vi "LabVIEWWebsocketChart - Multiple Connection.vi"() -> ()   [LabVIEW 2014]
uses:
  Modules/Library/Method.ctl
  <vilib>/myRIO/Instrument Drivers/Onboard IO/DIO/typedefs/DIO Reference.ctl
  <vilib>/myRIO/Common/Instrument Driver Framework/Utilities/typedefs/myRIO Generic Hardware Reference.ctl
  <vilib>/myRIO/Common/Instrument Driver Framework/Utilities/typedefs/Hardware Version Enum.ctl
  <vilib>/myRIO/Common/Instrument Driver Framework/Utilities/typedefs/myRIO v1.0 Reference.ctl
  <vilib>/myRIO/Common/Instrument Driver Framework/Utilities/typedefs/Generic FPGA Reference.ctl
  <vilib>/myRIO/Common/Instrument Driver Framework/myRIO v1.0/DIO/typedefs/DIO Channels List.ctl
  <vilib>/myRIO/Common/Instrument Driver Framework/myRIO v1.0/DIO/typedefs/DIO Channels Enum.ctl
  <vilib>/userdefined/High Color/nirio_resource_hc.ctl
  Modules/Library/Connection.ctl
  <vilib>/NI/STM/SubVIs/MetaDataElement.ctl
  <vilib>/myRIO/Instrument Drivers/Onboard Devices/Accelerometer/typedefs/Accelerometer Reference.ctl
  <vilib>/myRIO/Common/Instrument Driver Framework/myRIO v1.0/Accelerometer/typedefs/Accelerometer Channels List.ctl
  <vilib>/myRIO/Common/Instrument Driver Framework/myRIO v1.0/Accelerometer/typedefs/Accelerometer Channels Enum.ctl
  <vilib>/myRIO/Common/Instrument Driver Framework/Utilities/vis/Is FPGA Ref Available.vi
  <vilib>/myRIO/Common/Instrument Driver Framework/myRIO v1.0/DIO/vis/myRIO v1.1 Open DIO.vi
  <vilib>/myRIO/Instrument Drivers/Onboard IO/DIO/vis/Read.vi
  <vilib>/myRIO/Common/Instrument Driver Framework/myRIO v1.0/Accelerometer/vis/myRIO v1.1 Open Accelerometer.vi
  <vilib>/myRIO/Instrument Drivers/Onboard Devices/Accelerometer/vis/Read.vi
  <vilib>/myRIO/Instrument Drivers/Onboard IO/DIO/vis/Write.vi
  <vilib>/myRIO/Common/Instrument Driver Framework/Utilities/vis/Validate Channels.vi
  <vilib>/myRIO/Common/Instrument Driver Framework/myRIO v1.0/DIO/vis/myRIO v1.0 Reserve DIO.vi
  <vilib>/myRIO/Common/Instrument Driver Framework/myRIO v1.0/Accelerometer/vis/myRIO v1.0 Reserve Accelerometer.vi
  <vilib>/myRIO/Common/Instrument Driver Framework/myRIO v1.0/Resource Manager/vis/myRIO v1.0 Reserve Channel List.vi
  <vilib>/myRIO/Common/Instrument Driver Framework/myRIO v1.0/DIO/vis/myRIO v1.0 Build MUX Configuration DIO.vi
  <vilib>/myRIO/Common/Instrument Driver Framework/myRIO v1.0/Accelerometer/vis/myRIO v1.0 Build MUX Configuration Accelerometer.vi
  <vilib>/myRIO/Common/Instrument Driver Framework/myRIO v1.0/Resource Manager/vis/myRIO v1.0 Reserve Channel.vi
  <vilib>/myRIO/Common/Instrument Driver Framework/myRIO v1.0/Resource Manager/vis/myRIO v1.0 Unreserve Channel.vi
  <vilib>/myRIO/Common/Instrument Driver Framework/myRIO v1.0/Resource Manager/vis/myRIO v1.0 Create Configuration List.vi
  <vilib>/myRIO/Common/Instrument Driver Framework/myRIO v1.0/Resource Manager/vis/myRIO v1.0 Build Mutex Name.vi
  <vilib>/Utility/VariantDataType/GetNumericInfo.vi
  <vilib>/Utility/error.llb/Error Cluster From Error Code.vi
  <vilib>/myRIO/Common/Instrument Driver Framework/myRIO v1.0/myRIO v1.1 Open.vi
  <vilib>/myRIO/Common/Instrument Driver Framework/Utilities/vis/IO Manager.vi
  <vilib>/myRIO/Common/Instrument Driver Framework/Utilities/vis/Configuration Manager.vi
  <vilib>/myRIO/Common/Instrument Driver Framework/myRIO v1.0/Resource Manager/vis/myRIO v1.0 Configure IO.vi
  <vilib>/myRIO/Common/Instrument Driver Framework/myRIO v1.0/myRIO v1.0 Close.vi
  <vilib>/myRIO/Common/Instrument Driver Framework/myRIO v1.0/DIO/vis/myRIO v1.0 Read DIO.vi
  <vilib>/functionblocks/Edge Detection/One Shot Rising with Input/One Shot Rising with Input.vi
  <vilib>/myRIO/Common/Instrument Driver Framework/myRIO v1.0/DIO/vis/myRIO v1.0 Write DIO.vi
  <vilib>/myRIO/Common/Instrument Driver Framework/myRIO v1.0/Accelerometer/vis/myRIO v1.0 Get Scaling Constant Accelerometer.vi
  <vilib>/myRIO/Common/Instrument Driver Framework/myRIO v1.0/Accelerometer/vis/myRIO v1.0 Read Accelerometer.vi
  <vilib>/myRIO/Express VI/Onboard Devices/Button/Button Express VI.xnode
  <vilib>/myRIO/Instrument Drivers/Onboard IO/DIO/vis/myRIO DIO Open.xnode
  <vilib>/functionblocks/FB Core/FB Core.xnode
  <vilib>/myRIO/Express VI/Onboard Devices/LED/LED Express VI.xnode
  <vilib>/myRIO/Express VI/Onboard Devices/Accelerometer/Accelerometer Express VI.xnode
  <vilib>/myRIO/Instrument Drivers/Onboard Devices/Accelerometer/vis/myRIO Accelerometer Open.xnode
  <vilib>/Intelligent Energy/WebSockets API/WebSockets/WebSockets.lvlib
  <vilib>/NI/STM/NI STM.lvlib
  <vilib>/myRIO/Instrument Drivers/Onboard IO/DIO/DIO.lvlib
  <vilib>/functionblocks/NI_FunctionBlock Libraries.lvlib
  <vilib>/myRIO/Instrument Drivers/Onboard Devices/Accelerometer/Accelerometer.lvlib
panel:
  out "Chart":T1(graph)
  out "LED 2":bool
  out "LED 1":bool
  out "User Text (Log)":string="\r\n"
  out "User Text (Last)":string
  out "data (default)":string
  out "msg (default)":string="ssssss"
  out "data (JSON) 2":string
  out "msg (string)":string="Core : CN Close"
  in  "Toggle LED 2":bool
  in  "Toggle LED 1":bool
  out "Request URI":string="/"
  out "HTTP Headers":variant=variant("Accept"=variant(string "text/html,application/xhtml+xml,application/xml;q=0.9,*/*;q=0.8"), "Accept-Encoding"=variant(string "gzip, deflate"), "Accept-Language"=variant(string "en-GB,en;q=0.5"), "Cache-Control"=variant(string "no-cache"), "Connection"=variant(string "keep-alive, Upgrade"), "DNT"=variant(string "1"), "Host"=variant(string "localhost:6125"), "Origin"=variant(string "http://localhost:8000"), "Pragma"=variant(string "no-cache"), "Sec-WebSocket-Extensions"=variant(string "permessage-deflate"), "Sec-WebSocket-Key"=variant(string "dPMfcRTFpHjstnxySTdG7A=="), "Sec-WebSocket-Version"=variant(string "13"), "Upgrade"=variant(string "websocket"), "User-Agent"=variant(string "Mozilla/5.0 (Windows NT 10.0; WOW64; rv:42.0) Gecko/20100101 Firefox/42.0"))
  in  "Stop":bool
  in  "Send":bool
  in  "Message":string="new message"
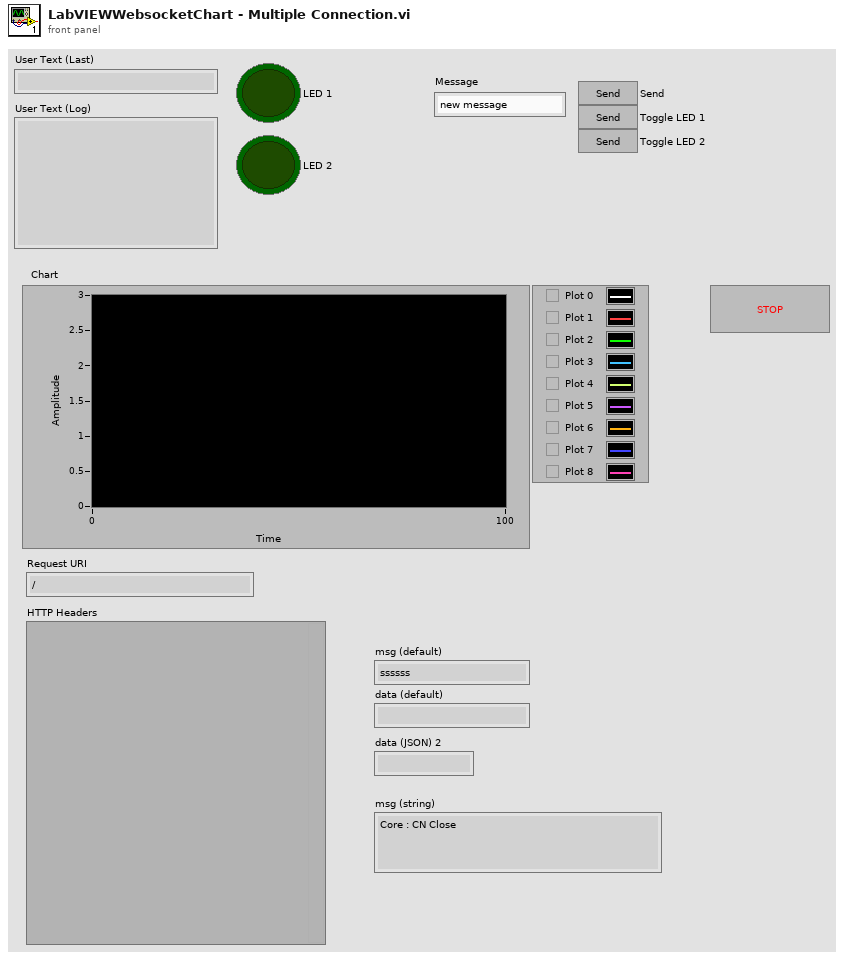
[diagram p1: front panel]
types:
  T1 = cluster{"[0]":dbl, "[1]":dbl, "[2]":dbl, "[3]":dbl, "[4]":dbl, "[5]":dbl, "[6]":dbl, "[7]":dbl, "[8]":dbl}
  T2 = typedef "Method.ctl" = enum16{"Initialize", "Add Connection", "Set Properties", "Get Connection(s)", "Remove Connection", "Remove All Connections", "Get Connection Count"}
  T3 = typedef "DIO.lvlib/DIO Reference.ctl" = cluster{"myRIO Reference":T4, "DIO Channels List":T8}
  T4 = typedef "myRIO Generic Hardware Reference.ctl" = cluster{"myRIO Model":T5, "myRIO Hardware Reference":T6}
  T5 = typedef "Hardware Version Enum.ctl" = enum16{"Unknown", "myRIO-1900", "myRIO-1950"}
  T6 = typedef "myRIO v1.0 Reference.ctl" = cluster{"Generic FPGA Reference":T7, "Allow multiple opens":bool}
  T7 = typedef "Generic FPGA Reference.ctl" = refnum<k20>
  T8 = typedef "DIO Channels List.ctl" = T9[]
  T9 = typedef "DIO Channels Enum.ctl" = enum16{"Not Connected", "C/DIO0", "C/DIO1", "C/DIO2", "C/DIO3", "C/DIO4", "C/DIO5", "C/DIO6", "C/DIO7", "A/DIO0", "A/DIO1", "A/DIO2", "A/DIO3", "A/DIO4", "A/DIO5", "A/DIO6", "A/DIO7", "A/DIO8", "A/DIO9", "A/DIO10", "A/DIO11", "A/DIO12", "A/DIO13", "A/DIO14", "A/DIO15", "B/DIO0", "B/DIO1", "B/DIO2", "B/DIO3", "B/DIO4", "B/DIO5", "B/DIO6", "B/DIO7", "B/DIO8", "B/DIO9", "B/DIO10", "B/DIO11", "B/DIO12", "B/DIO13", "B/DIO14", "B/DIO15", "LED0", "LED1", "LED2", "LED3", "Button0"}
  T10 = typedef "nirio_resource_hc.ctl" = tag
  T11 = typedef "NI STM.lvlib/TCP Connection Info.ctl" = cluster{"connection ID":refnum<k5>, "meta data":T12[]}
  T12 = typedef "NI STM.lvlib/MetaDataElement.ctl" = string
  T13 = typedef "Connection.ctl" = cluster{"connection ID":refnum<k5>, "meta data":T12[]}
  T14 = typedef "Accelerometer.lvlib/Accelerometer Reference.ctl" = cluster{"myRIO Reference":T4, "Accelerometer Channels List":T15, "LSB Weight":dbl}
  T15 = typedef "Accelerometer Channels List.ctl" = T16[]
  T16 = typedef "Accelerometer Channels Enum.ctl" = enum16{"Not Connected", "X-Axis", "Y-Axis", "Z-Axis"}
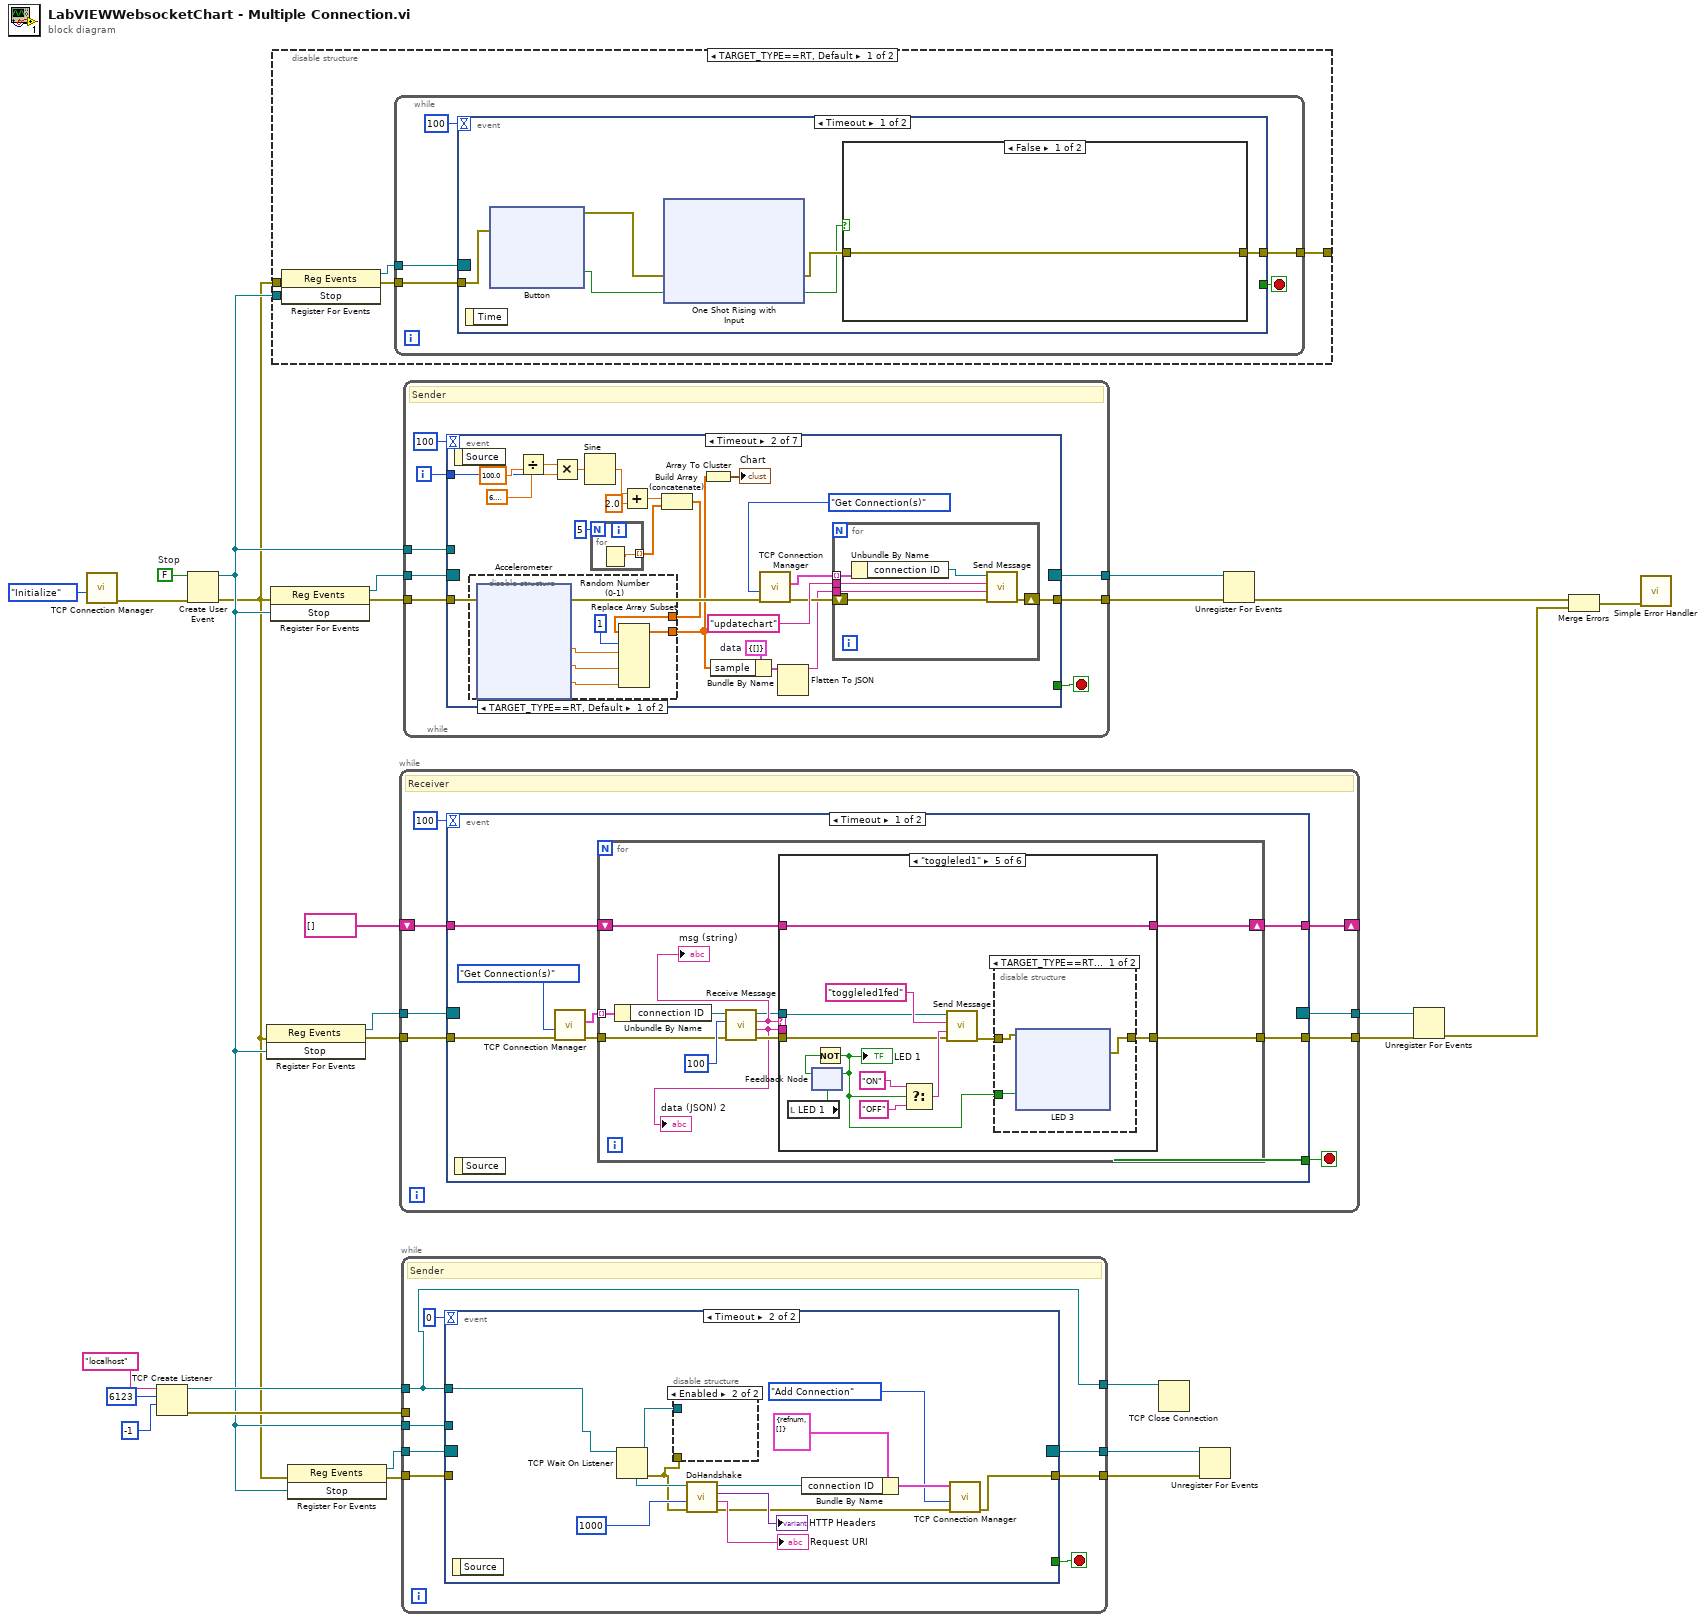
[diagram p0: block diagram]
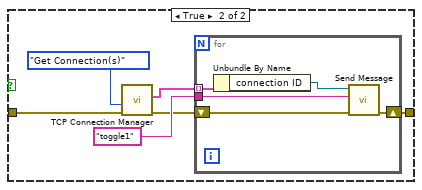
[diagram p2: hidden frame]
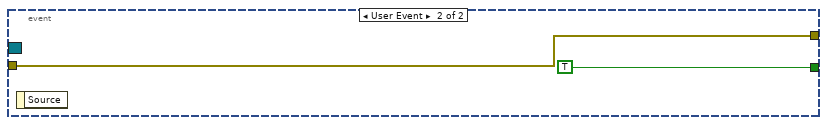
[diagram p3: hidden frame]
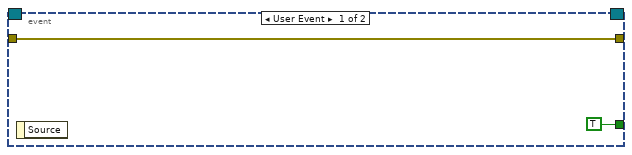
[diagram p5: hidden frame]
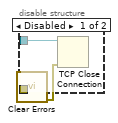
[diagram p6: hidden frame]
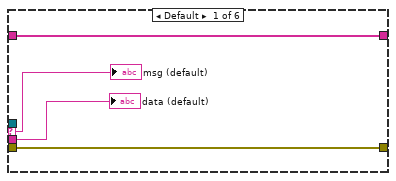
[diagram p7: hidden frame]
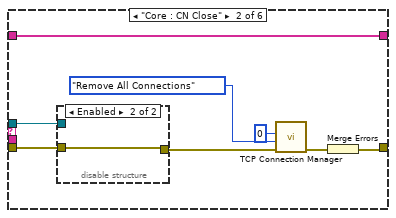
[diagram p8: hidden frame]
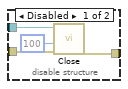
[diagram p9: hidden frame]
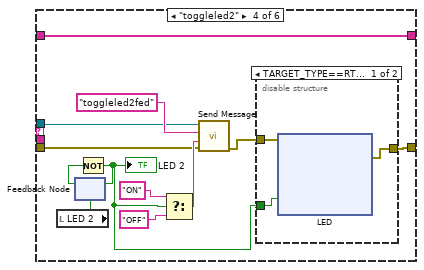
[diagram p11: hidden frame]
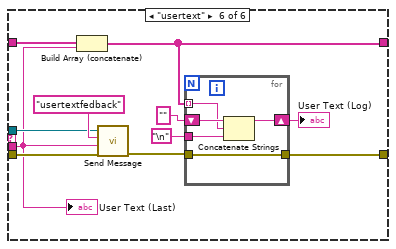
[diagram p14: hidden frame]
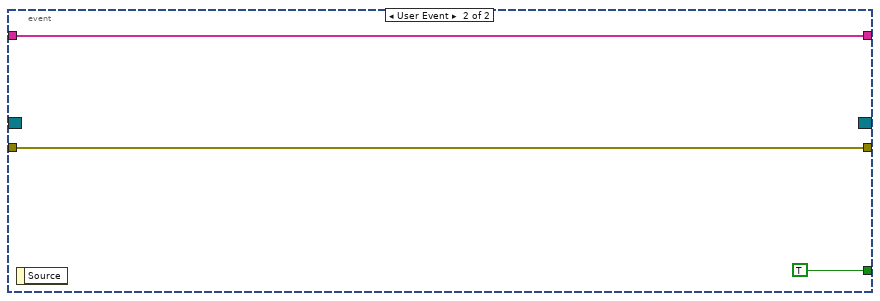
[diagram p15: hidden frame]
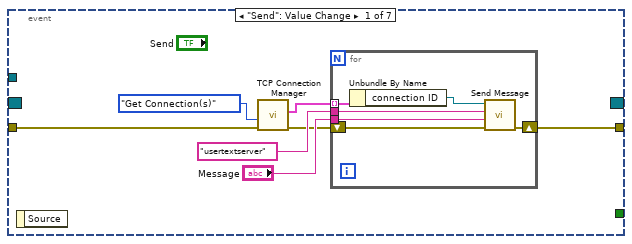
[diagram p16: hidden frame]
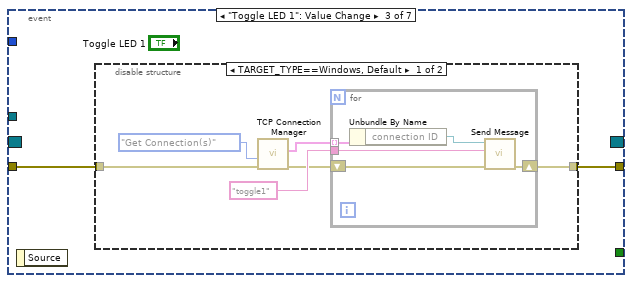
[diagram p18: hidden frame]
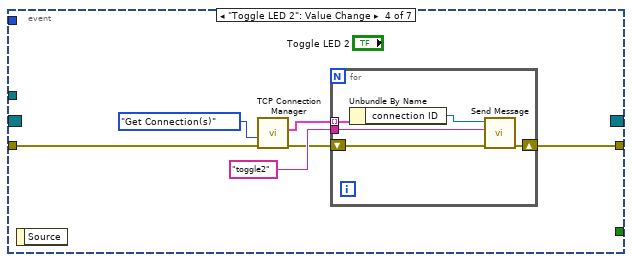
[diagram p20: hidden frame]
diagram:
  w27 = FALSE  # Stop
  n1 = call "TCP Connection Manager.vi"("method"=Method."Initialize") -> ("error out"=w10:errorcluster)  [unwired: 7 in, 3 out]
  n2 = TCP Create Listener(9:-1 ("timeout ms (25000)"), 10:u16 6123 ("port"), 11:"localhost" ("service name")) -> (0:w3:errorcluster, 3:w5:refnum<k5>)  [unwired: 2 in, 1 out]
  n3 = Create User Event(user event datatype=w27, error in=w10) -> (user event=w2:refnum<user-event>, error out=w1:errorcluster)
  n4 = register-events(error in=w1, w2) -> (reference out=w20:refnum<event-registration>, error out=w19:errorcluster)  [unwired: 1 in]
  n5 = register-events(error in=w1, w2) -> (reference out=w25:refnum<event-registration>, error out=w26:errorcluster)  [unwired: 1 in]
  n6 = disable-structure shown="TARGET_TYPE==RT, Default" {
    disable-tunnel: w2 -> [w31 _]
    disable-tunnel: w1 -> [w30 _]
    disable-tunnel: [w28 _] -> _
    frame condition #0 (active) {
      n7 = register-events(error in=w30, w31) -> (reference out=w29:refnum<event-registration>, error out=w32:errorcluster)  [unwired: 1 in]
      n8 = while {
        tunnel: w32 -> [w36]
        tunnel: w29 -> [w35]
        tunnel: [w33] -> w28
        stop <- w34 stop-if-true
        n9 = event shown="[0] Timeout" {
          selector: w35 -> [_ _]
          dyn-events: _ -> [_ _]
          timeout: 100 -> [_ _]
          tunnel: w36 -> [w42 w129]
          tunnel: [_ TRUE] -> w34
          tunnel: [w43 w129] -> w33
          event Timeout {
            n10 = event-data() -> ()  [unwired: 1 in, 1 out]
            n11 = xnode "Button"("error in (no error)"=w42) -> ("Value"=w40:bool, "error out"=w41:errorcluster)
            n12 = xnode "One Shot Rising with Input"("error in"=w41, "input"=w40) -> ("error out"=w39:errorcluster, "output"=w38:bool)
            n13 = case shown="False" w38 {
              tunnel: w39 -> [w117 w119]
              tunnel: [w117 w118] -> w43
              frame False {
              }
              frame True {
                n14 = call "TCP Connection Manager.vi"("error in"=w119, "method"=Method."Get Connection(s)") -> ("error out"=w122:errorcluster, "all connections"=w120:T11[])  [unwired: 6 in, 2 out]
                n15 = for {
                  tunnel: "toggle1" ("msg (string)") -> [w128]
                  tunnel: w120 -> [w126] mode=indexing
                  shift-right: [w124] -> w118
                  shift-left: w122 -> [w127]
                  n16 = Unbundle By Name(w126) -> ("connection ID"=w125:refnum<k5>)
                  n17 = call "Send Message.vi"("error in (no error)"=w127, "msg (string)"=w128, "WebSocket Connection in"=w125) -> ("error out"=w124:errorcluster)  [unwired: 7 in, 1 out]
                }
              }
            }
          }
          event User Event {
            n18 = event-data() -> ()  [unwired: 1 in, 1 out]
          }
        }
      }
    }
    frame condition #1 {
    }
  }
  n19 = register-events(error in=w1, w2) -> (reference out=w13:refnum<event-registration>, error out=w14:errorcluster)  [unwired: 1 in]
  n20 = while {
    tunnel: w20 -> [w136]
    tunnel: [w134] -> w22
    shift-right: [w131] -> _
    shift-left: string[] [] ("appended array") -> [w132]
    tunnel: w19 -> [w135]
    tunnel: [w137] -> w21
    stop <- w138 stop-if-true
    # "Receiver"
    n21 = event shown="[0] Timeout" {
      selector: w136 -> [_ _]
      dyn-events: [_ _] -> w134
      timeout: 100 -> [_ _]
      tunnel: [_ TRUE] -> w138
      tunnel: [w142 w295] -> w137
      tunnel: w135 -> [w145 w295]
      tunnel: w132 -> [w141 w294]
      tunnel: [w140 w294] -> w131
      event Timeout {
        n22 = event-data() -> ()  [unwired: 1 in, 1 out]
        n23 = call "TCP Connection Manager.vi"("error in"=w145, "method"=Method."Get Connection(s)") -> ("error out"=w143:errorcluster, "all connections"=w139:T11[])  [unwired: 6 in, 2 out]
        n24 = for {
          tunnel: w143 -> [w155]
          tunnel: [w151] -> w142
          tunnel: w139 -> [w154] mode=indexing
          shift-right: [w149] -> w140
          shift-left: w141 -> [w150]
          n25 = Unbundle By Name(w154) -> ("connection ID"=w153:refnum<k5>)
          n26 = call "Receive Message.vi"("error in (no error)"=w155, "timeout ms (5000)"=100, "WebSocket Connection in"=w153) -> ("error out"=w152:errorcluster, "data (JSON)"=w147:string, "msg (string)"=w148:string, "WebSocket Connection out"=w146:refnum<k5>)  [unwired: 5 in]
          "msg (string)" <- w148
          "data (JSON) 2" <- w147
          n27 = case shown="\"toggleled1\"" w148 {
            selector: w148 -> [w159 _ _ _ _ _]
            tunnel: w152 -> [w160 w167 w174 w181 w232 w286]
            tunnel: w147 -> [w158 _ _ _ _ w284]
            tunnel: [w160 w165 w174 w178 w228 w280] -> w151
            tunnel: w150 -> [w157 w168 w175 w180 w231 w288]
            tunnel: [w157 w168 w175 w180 w231 w278] -> w149
            tunnel: w146 -> [_ w166 _ w179 w230 w285]
            frame Default {
              "msg (default)" <- w159
              "data (default)" <- w158
            }
            frame "Core : CN Close" {
              n28 = disable-structure shown="Enabled" {
                disable-tunnel: w167 -> [w172 w173]
                disable-tunnel: w166 -> [w171 _]
                disable-tunnel: [w169 w173] -> w162
                frame Disabled {
                  n29 = call <vilib>:"Close.vi"("error in (no error)"=w172, "timeout ms (5000)"=100, "WebSocket Connection in"=w171) -> ("error out"=w169:errorcluster)  [unwired: 7 in, 1 out]
                }
                frame Enabled {
                }
              }
              n30 = call "TCP Connection Manager.vi"("error in"=w162, "method"=Method."Remove All Connections", "index"=0) -> ("error out"=w164:errorcluster)  [unwired: 5 in, 3 out]
              n31 = Merge Errors(w164) -> (w165:errorcluster)
            }
            frame "Core :Timeout" {
            }
            frame "toggleled2" {
              n32 = local read "LED 2"() -> (w182:bool)
              n33 = feedback #1(w182) -> (w183:bool)
              n34 = Not(x=w183) -> (.not. x?=w176:bool)
              "LED 2" <- w176
              n35 = feedback-in #1(w176) -> ()
              n36 = Select(t="ON", s=w176, f="OFF") -> (s? t:f=w187:string)
              n37 = call "Send Message.vi"("error in (no error)"=w181, "data (JSON)"=w187, "msg (string)"="toggleled2fed", "WebSocket Connection in"=w179) -> ("error out"=w177:errorcluster)  [unwired: 6 in, 1 out]
              n38 = disable-structure shown="TARGET_TYPE==RT, Default" {
                disable-tunnel: w177 -> [w190 w226]
                disable-tunnel: [w189 w226] -> w178
                disable-tunnel: w176 -> [w188 _]
                frame condition #0 (active) {
                  n39 = xnode "LED"("LED1"=w188, "error in (no error)"=w190) -> ("error out"=w189:errorcluster)
                }
                frame condition #1 {
                }
              }
            }
            frame "toggleled1" {
              n40 = local read "LED 1"() -> (w233:bool)
              n41 = feedback #2(w233) -> (w234:bool)
              n42 = Not(x=w234) -> (.not. x?=w227:bool)
              "LED 1" <- w227
              n43 = feedback-in #2(w227) -> ()
              n44 = Select(t="ON", s=w227, f="OFF") -> (s? t:f=w238:string)
              n45 = call "Send Message.vi"("error in (no error)"=w232, "data (JSON)"=w238, "msg (string)"="toggleled1fed", "WebSocket Connection in"=w230) -> ("error out"=w229:errorcluster)  [unwired: 6 in, 1 out]
              n46 = disable-structure shown="TARGET_TYPE==RT, Default" {
                disable-tunnel: w229 -> [w241 w277]
                disable-tunnel: [w240 w277] -> w228
                disable-tunnel: w227 -> [w239 _]
                frame condition #0 (active) {
                  n47 = xnode "LED 3"("LED0"=w239, "error in (no error)"=w241) -> ("error out"=w240:errorcluster)
                }
                frame condition #1 {
                }
              }
            }
            frame "usertext" {
              n48 = Build Array (concatenate)(w288, w284) -> (w278:string[])
              n49 = call "Send Message.vi"("error in (no error)"=w286, "data (JSON)"=w284, "msg (string)"="usertextfedback", "WebSocket Connection in"=w285) -> ("error out"=w279:errorcluster)  [unwired: 6 in, 1 out]
              n50 = for {
                tunnel: w278 -> [w291] mode=indexing
                shift-right: [w293] -> w282
                shift-left: "" -> [w292]
                tunnel: "\n" -> [w290]
                tunnel: w279 -> [w289]
                tunnel: [w289] -> w280
                n51 = Concatenate Strings(w292, w291, w290) -> (w293:string)
              }
              "User Text (Log)" <- w282
              "User Text (Last)" <- w284
            }
          }
        }
      }
      event User Event {
        n52 = event-data() -> ()  [unwired: 1 in, 1 out]
      }
    }
  }
  n53 = while {
    tunnel: w13 -> [w302]
    tunnel: [w300] -> w11
    tunnel: w2 -> [w299]
    tunnel: w14 -> [w301]
    tunnel: [w303] -> w12
    tunnel: w5 -> [w297]
    tunnel: [w297] -> w4
    tunnel: w3 -> [_]
    stop <- w304 stop-if-true
    # "Sender"
    n54 = event shown="[1] Timeout" {
      selector: w302 -> [_ _]
      dyn-events: [_ _] -> w300
      timeout: 0 -> [_ _]
      tunnel: [TRUE _] -> w304
      tunnel: [w305 w319] -> w303
      tunnel: w301 -> [w305 _]
      tunnel: w299 -> [_ _]
      tunnel: w297 -> [_ w307]
      event User Event {
        n55 = event-data() -> ()  [unwired: 1 in, 1 out]
      }
      event Timeout {
        n56 = event-data() -> ()  [unwired: 1 in, 1 out]
        n57 = TCP Wait On Listener(11:w307) -> (0:w308:errorcluster, 3:w309:refnum<k5>, 4:w315:refnum<k5>)  [unwired: 3 in, 2 out]
        n58 = disable-structure shown="Enabled" {
          disable-tunnel: w309 -> [w322 _]
          disable-tunnel: w308 -> [w321 _]
          frame Disabled {
            n59 = call <vilib>:"Clear Errors.vi"("error in (no error)"=w321) -> ("error out"=w320:errorcluster)  [unwired: 5 in, 1 out]
            n60 = TCP Close Connection(connection ID=w322, error in (no error)=w320) -> ()  [unwired: 1 in, 2 out]
          }
          frame Enabled {
          }
        }
        n61 = call <vilib>:"DoHandshake.vi"("error in (no error)"=w308, "timeout ms (5000)"=1000 ("timeout ms (25000)"), "WebSocket Connection in"=w315) -> ("error out"=w312:errorcluster, "Request URI"=→"Request URI":string, "Headers Out"=→"HTTP Headers":variant, "WebSocket Connection out"=w313:refnum<k5>)  [unwired: 5 in]
        n62 = Bundle By Name(cluster=T13 {"connection ID"=refnum, "meta data"=[]} ("connection in"), "connection ID"=w313) -> (w311:T13)
        n63 = call "TCP Connection Manager.vi"("error in"=w312, "method"=Method."Add Connection", "connection in"=w311) -> ("error out"=w319:errorcluster)  [unwired: 5 in, 3 out]
      }
    }
  }
  n64 = while {
    tunnel: w25 -> [w328]
    tunnel: [w326] -> w23
    tunnel: w2 -> [w325]
    tunnel: w26 -> [w327]
    tunnel: [w329] -> w24
    i -> [w323]
    stop <- w330 stop-if-true
    # "Sender"
    n65 = event shown="[1] Timeout" {
      selector: w328 -> [_ _ _ _ _ _ _]
      dyn-events: [_ _ _ _ _ _ _] -> w326
      timeout: 100 -> [_ _ _ _ _ _ _]
      tunnel: [_ _ _ _ FALSE _ TRUE] -> w330
      tunnel: [w334 w363 w420 w436 w445 w451 w454] -> w329
      tunnel: w327 -> [w333 w362 w419 w435 w447 w453 w454]
      tunnel: w325 -> [_ _ _ _ w446 w452 _]
      tunnel: w323 -> [_ w351 _ _ _ _ _]
      event "Send": Value Change {
        n66 = event-data() -> ()  [unwired: 1 in, 1 out]
        n67 = call "TCP Connection Manager.vi"("error in"=w333, "method"=Method."Get Connection(s)") -> ("error out"=w335:errorcluster, "all connections"=w331:T11[])  [unwired: 6 in, 2 out]
        n68 = for {
          tunnel: "usertextserver" ("msg (string)") -> [w343]
          tunnel: "Message" -> [w342]
          tunnel: w331 -> [w340] mode=indexing
          shift-right: [w338] -> w334
          shift-left: w335 -> [w341]
          n69 = Unbundle By Name(w340) -> ("connection ID"=w339:refnum<k5>)
          n70 = call "Send Message.vi"("error in (no error)"=w341, "data (JSON)"=w342, "msg (string)"=w343, "WebSocket Connection in"=w339) -> ("error out"=w338:errorcluster)  [unwired: 6 in, 1 out]
        }
      }
      event Timeout {
        w350 = cluster{"sample":dbl[]} {"sample"=[]}  # data
        n71 = event-data() -> ()  [unwired: 1 in, 1 out]
        n72 = Divide(x=w351, y=100.0) -> (x/y=w357:dbl)
        n73 = Multiply(x=w357, y=6.283185307179586) -> (x*y=w358:dbl)
        n74 = Sine(x=w358) -> (sin(x)=w360:dbl)
        n75 = for {
          N: 5 -> [_]
          tunnel: [w412] -> w353 mode=indexing
          n76 = Random Number (0-1)() -> (number: 0 to 1=w412:dbl)
        }
        n77 = Add(x=w360, y=2.0) -> (x+y=w354:dbl)
        n78 = Build Array (concatenate)(w354, w353) -> (w345:dbl[])
        n79 = disable-structure shown="TARGET_TYPE==RT, Default" {
          disable-tunnel: w345 -> [w371 w411]
          disable-tunnel: [w370 w411] -> w344
          frame condition #0 (active) {
            n80 = xnode "Accelerometer"() -> ("X-Axis"=w368:dbl, "Y-Axis"=w367:dbl, "Z-Axis"=w366:dbl)  [unwired: 1 in, 1 out]
            n81 = Replace Array Subset(array=w371, new element #1=w368, index #1=1 ("index"), new element #2=w367, new element #3=w366) -> (w370:dbl[])  [unwired: 2 in]
          }
          frame condition #1 {
          }
        }
        n82 = Array To Cluster(array=w344) -> (cluster=→"Chart":T1)
        n83 = Bundle By Name(cluster=w350, "sample"=w344) -> (w349:cluster{"sample":dbl[]})
        n84 = call "TCP Connection Manager.vi"("error in"=w362, "method"=Method."Get Connection(s)") -> ("error out"=w364:errorcluster, "all connections"=w347:T11[])  [unwired: 6 in, 2 out]
        n85 = Flatten To JSON(anything=w349) -> (JSON string=w348:string)  [unwired: 2 in, 1 out]
        n86 = for {
          tunnel: "updatechart" ("msg (string)") -> [w418]
          tunnel: w348 -> [w417]
          tunnel: w347 -> [w415] mode=indexing
          shift-right: [w413] -> w363
          shift-left: w364 -> [w416]
          n87 = Unbundle By Name(w415) -> ("connection ID"=w414:refnum<k5>)
          n88 = call "Send Message.vi"("error in (no error)"=w416, "data (JSON)"=w417, "msg (string)"=w418, "WebSocket Connection in"=w414) -> ("error out"=w413:errorcluster)  [unwired: 6 in, 1 out]
        }
      }
      event "Toggle LED 1": Value Change {
        n89 = event-data() -> ()  [unwired: 1 in, 1 out]
        n90 = disable-structure shown="TARGET_TYPE==Windows, Default" {
          disable-tunnel: [w424 w432] -> w420
          disable-tunnel: w419 -> [w423 w432]
          frame condition #0 {
            n91 = call "TCP Connection Manager.vi"("error in"=w423, "method"=Method."Get Connection(s)") -> ("error out"=w425:errorcluster, "all connections"=w421:T11[])  [unwired: 6 in, 2 out]
            n92 = for {
              tunnel: "toggle1" ("msg (string)") -> [w431]
              tunnel: w421 -> [w429] mode=indexing
              shift-right: [w427] -> w424
              shift-left: w425 -> [w430]
              n93 = Unbundle By Name(w429) -> ("connection ID"=w428:refnum<k5>)
              n94 = call "Send Message.vi"("error in (no error)"=w430, "msg (string)"=w431, "WebSocket Connection in"=w428) -> ("error out"=w427:errorcluster)  [unwired: 7 in, 1 out]
            }
          }
          frame condition #1 (active) {
          }
        }
      }
      event "Toggle LED 2": Value Change {
        n95 = event-data() -> ()  [unwired: 1 in, 1 out]
        n96 = call "TCP Connection Manager.vi"("error in"=w435, "method"=Method."Get Connection(s)") -> ("error out"=w437:errorcluster, "all connections"=w433:T11[])  [unwired: 6 in, 2 out]
        n97 = for {
          tunnel: "toggle2" ("msg (string)") -> [w443]
          tunnel: w433 -> [w441] mode=indexing
          shift-right: [w439] -> w436
          shift-left: w437 -> [w442]
          n98 = Unbundle By Name(w441) -> ("connection ID"=w440:refnum<k5>)
          n99 = call "Send Message.vi"("error in (no error)"=w442, "msg (string)"=w443, "WebSocket Connection in"=w440) -> ("error out"=w439:errorcluster)  [unwired: 7 in, 1 out]
        }
      }
      event "Stop": Value Change {
        n100 = event-data() -> ()  [unwired: 1 in, 1 out]
        n101 = Generate User Event(user event=w446, event data cluster=TRUE ("event data"), error in=w447) -> (error out=w445:errorcluster)  [unwired: 1 in, 1 out]
      }
      event Panel Close? {
        n102 = event-data() -> ()  [unwired: 1 in, 1 out]
        n103 = Generate User Event(user event=w452, event data cluster=TRUE ("event data"), error in=w453) -> (error out=w451:errorcluster)  [unwired: 1 in, 1 out]
        n104 = event-data("Discard?"=TRUE) -> ()  [unwired: 1 in, 1 out]
      }
      event User Event {
        n105 = event-data() -> ()  [unwired: 1 in, 1 out]
      }
    }
  }
  n106 = TCP Close Connection(connection ID=w4) -> ()  [unwired: 2 in, 2 out]
  n107 = Unregister For Events(event registration refnum=w11, error in=w12) -> ()  [unwired: 1 out]
  n108 = Unregister For Events(event registration refnum=w23, error in=w24) -> (error out=w17:errorcluster)
  n109 = Unregister For Events(event registration refnum=w22, error in=w21) -> (error out=w16:errorcluster)
  n110 = Merge Errors(w17, w16) -> (w15:errorcluster)
  n111 = call <vilib>:"Simple Error Handler.vi"("error in (no error)"=w15) -> ()  [unwired: 4 in, 5 out]
